vi "Analyze_ROI_Image.vi"(0 "ImageIn":T2(plugin-control), 1 "ProjectName":string, 2 "ForCalCalculaton In":T2, 5 "ROI Entry":T4={"vROIName"="", "vROIContour"={"Contour Type"=0, "ROI Type"=0, "Points"=[]}, "ProcessSetting"=[], "Analysis_Setting"={"PreProcess"=enum."*Algorithm*", "Parameter"=""}}, 7 "Script Index":i32, 9 "Coordinate System In":T3 {"Measurement System"."Axis Reference" items=["Direct", "Indirect"]; "Measurement System"."Angle (deg)" format="%.2f"; "Measurement System"."Origin"."Y" format="%.2f"; "Measurement System"."Origin"."X" format="%.2f"; "Reference System"."Axis Reference" items=["Direct", "Indirect"]; "Reference System"."Angle (deg)" format="%.2f"; "Reference System"."Origin"."Y" format="%.2f"; "Reference System"."Origin"."X" format="%.2f"}, 11 "error in (no error)":errorcluster, 12 "RootPath":path, 13 "CreatDllImage":bool, 14 "Cam Index":i32) -> (4 "ExtractedProcessedImage":T2(plugin-control), 6 "AnalysisResult":variant, 8 "Analysis_Point_Result Out Overlay":T1[](array[typedef]), 10 "Analysis_Point_Result":T1[](array[typedef]), 15 "error out":errorcluster)   [LabVIEW 2019]
uses:
  <vilib>/vision/NI_Vision_Development_Module.lvlib
  DLL/[Global] ExtractedAnalizedImage.vi
  Process/Controls/Process_Setting.ctl
  Analysis/Controls/Analysis_Setting.ctl
  Controls/Vision_DataEntry.ctl
  Analysis/Controls/Analysis_Result_To_Caliper.ctl
  <vilib>/vision/Image Controls.llb/IMAQ Image.ctl
  Ctrl/VisionProcessName.ctl
panel:
  out "Image Type":T9 items=["Grayscale (U8)", "Grayscale (I16)", "Grayscale (SGL)", "Complex (CSG)", "RGB (U32)", "HSL (U32)", "RGB (U64)", "Grayscale (U16)"]
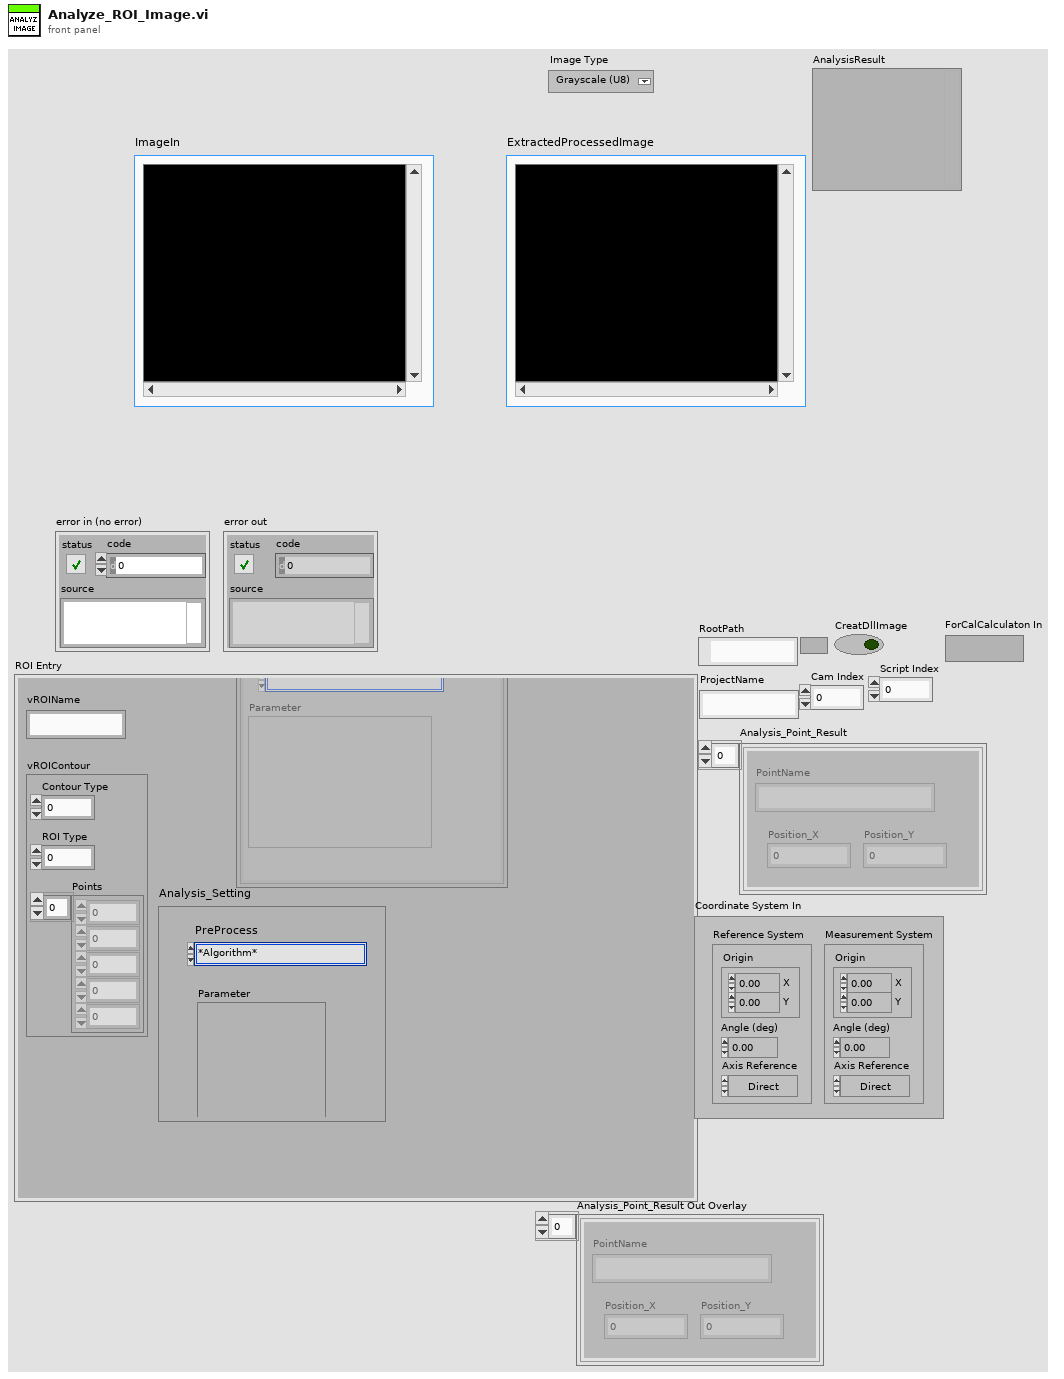
[diagram p1: front panel]
types:
  T1 = typedef "Analysis_Result_To_Caliper.ctl" = cluster{"PointName":string, "Position_X":dbl, "Position_Y":dbl}
  T2 = typedef "IMAQ Image.ctl" = refnum<image>
  T3 = cluster{"Reference System":cluster{"Origin":cluster{"X":sgl, "Y":sgl}, "Angle (deg)":sgl, "Axis Reference":u32}, "Measurement System":cluster{"Origin":cluster{"X":sgl, "Y":sgl}, "Angle (deg)":sgl, "Axis Reference":u32}}
  T4 = typedef "Vision_DataEntry.ctl" = cluster{"vROIName":string, "vROIContour":cluster{"Contour Type":u32, "ROI Type":u32, "Points":i32[]}, "ProcessSetting":T5[], "Analysis_Setting":T7}
  T5 = typedef "Process_Setting.ctl" = cluster{"Enum_PreProcess":T6, "Parameter":string}
  T6 = typedef "VisionProcessName.ctl" = enum16{"*CamParameter*", "CamAttributes", "*Preprocess*", "CG_Brightness", "C_Plane Extraction", "C_Threshold", "G_Lookup Table", "G_Threshold"}
  T7 = typedef "Analysis_Setting.ctl" = cluster{"PreProcess":T8, "Parameter":string}
  T8 = typedef "VisionProcessName.ctl" = enum16{"*CamParameter*", "CamAttributes", "*Preprocess*", "CG_Brightness", "C_Plane Extraction", "C_Threshold", "G_Lookup Table", "G_Threshold", "B_Image Inversion", "*Algorithm*", "CG_Histogram", "C_Color Matching", "C_Color Pattern Matching", "G_PatternMatch", "CG_Find Straight Edge", "CG_Adv. Find Straight Edge", "CG_Find Circular Edge", "G_Max Clamp", "G_Clamp (Rake)", "G_Pattern Matching"}
  T9 = typedef "Image Type" = u32
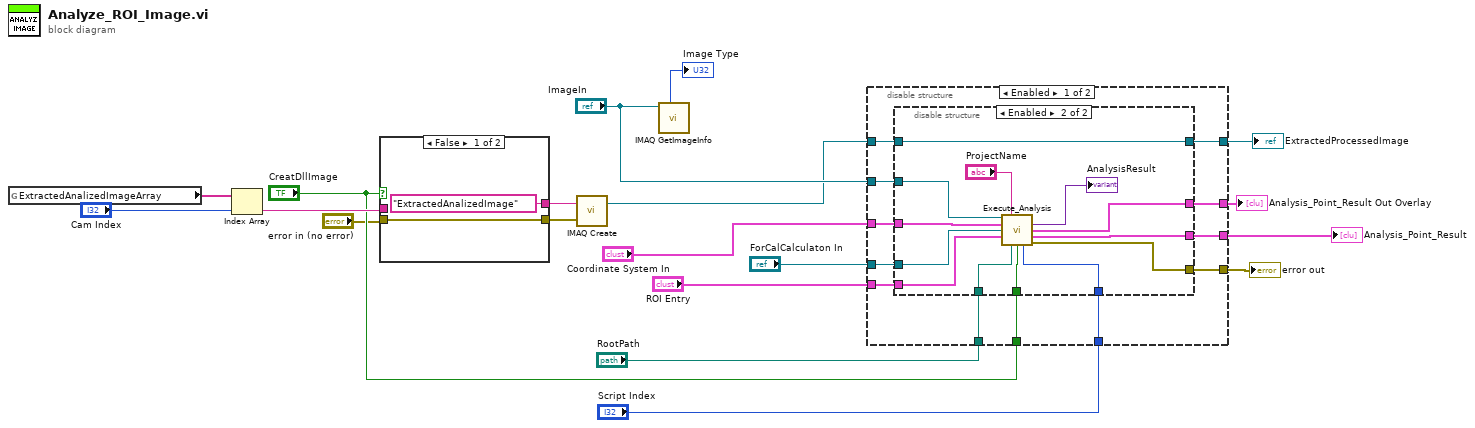
[diagram p0: block diagram]
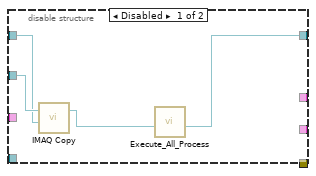
[diagram p3: hidden frame]
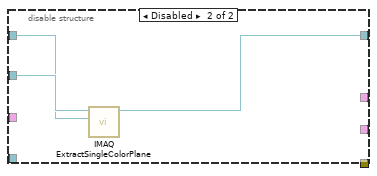
[diagram p4: hidden frame]
diagram:
  n1 = global read "[Global] ExtractedAnalizedImage.vi" "ExtractedAnalizedImageArray"() -> (w11:string[])
  n2 = Index Array(array=w11, index="Cam Index") -> (element=w10:string)
  n3 = case shown="False" "CreatDllImage" {
    tunnel: ["ExtractedAnalizedImage" ("Image Name") w23] -> w12
    tunnel: w10 -> [_ w23]
    tunnel: [w20 w22] -> w3
    tunnel: "error in (no error)" -> [w20 w22]
    frame False {
    }
    frame True {
    }
  }
  n4 = call "IMAQ Create"("Image Name"=w12, "error in (no error)"=w3) -> ("New Image"=w1:T2)  [unwired: 2 in, 2 out]
  n5 = call "IMAQ GetImageInfo"("Image"="ImageIn") -> ("Image Type"=→"Image Type":T9)  [unwired: 3 in, 7 out]
  n6 = disable-structure shown="Enabled" {
    disable-tunnel: "ImageIn" -> [w35 w56]
    disable-tunnel: [w33 w54] -> w18
    disable-tunnel: w1 -> [w34 w55]
    disable-tunnel: "ROI Entry" -> [w32 _]
    disable-tunnel: "RootPath" -> [w24 _]
    disable-tunnel: [w31 _] -> w14
    disable-tunnel: "Coordinate System In" -> [w30 _]
    disable-tunnel: "CreatDllImage" -> [w29 _]
    disable-tunnel: "Script Index" -> [w28 _]
    disable-tunnel: [w27 _] -> w7
    disable-tunnel: "ForCalCalculaton In" -> [w26 _]
    disable-tunnel: [w25 _] -> w5
    frame Enabled {
      n7 = disable-structure shown="Enabled" {
        disable-tunnel: w35 -> [w39 w53]
        disable-tunnel: w34 -> [w38 w52]
        disable-tunnel: [w36 w52] -> w33
        disable-tunnel: w32 -> [_ w50]
        disable-tunnel: w24 -> [_ w47]
        disable-tunnel: [_ w48] -> w31
        disable-tunnel: w30 -> [_ w46]
        disable-tunnel: w29 -> [_ w45]
        disable-tunnel: w28 -> [_ w44]
        disable-tunnel: [_ w43] -> w27
        disable-tunnel: w26 -> [_ w42]
        disable-tunnel: [_ w41] -> w25
        frame Disabled {
          n8 = call "IMAQ Copy"("Image Dst"=w38, "Image Src"=w39) -> ("Image Dst Out"=w37:T2)  [unwired: 4 in, 1 out]
          n9 = call "Execute_All_Process.vi"("ImageIn"=w37) -> ("Image Out"=w36:T2, "ProcessSettingIn"=w40:T5[])  [unwired: 4 in, 5 out]
        }
        frame Enabled {
          n10 = call "Execute_Analysis.vi"("Image In"=w53, "ProjectName"="ProjectName", "Coordinate System Out (Set Coordinate System 1)"=w46, "ForCalCalculaton In"=w42, "ROI Entry"=w50, "RootPath"=w47, "CreatDllImage"=w45, "Script Index"=w44) -> ("Result"=→"AnalysisResult":variant, "Analysis_Point_Result Out Overlay"=w41:T1[], "Analysis_Point_Result Out"=w48:T1[], "error out"=w43:errorcluster)  [unwired: 3 in, 1 out]
        }
      }
    }
    frame Disabled {
      n11 = call "IMAQ ExtractSingleColorPlane"("Image Dst"=w55, "Image Src"=w56) -> ("Image Dst Out"=w54:T2)  [unwired: 8 in, 1 out]
    }
  }
  "error out" <- w7
  "ExtractedProcessedImage" <- w18
  "Analysis_Point_Result" <- w14
  "Analysis_Point_Result Out Overlay" <- w5
